vi "Set Information.vi"(8 "error in (no error)":errorcluster, 10 "Inforamtion":string="Processing......", 11 "UI_ProgressBar in":refnum<class "UI_ProgressDlg.lvclass">) -> (0 "error out":errorcluster, 3 "UI_ProgressBar out":refnum<class "UI_ProgressDlg.lvclass">)   [LabVIEW 2014, in "UI_ProgressDlg.lvlib" / "UI_ProgressDlg.lvclass"]
uses:
  UI_ProgressDlg.lvclass
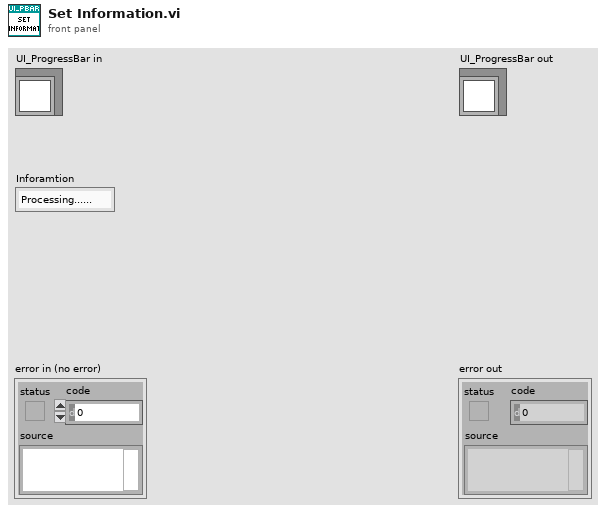
[diagram p1: front panel]
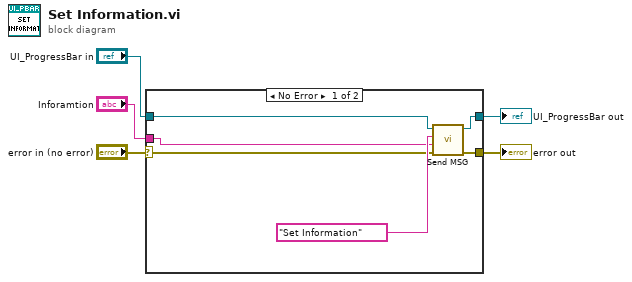
[diagram p0: block diagram]
diagram:
  n1 = case shown="No Error" "error in (no error)" {
    selector: "error in (no error)" -> [w6 w13]
    tunnel: [w10 w13] -> w4
    tunnel: [w11 w12] -> w2
    tunnel: "UI_ProgressBar in" -> [w9 w12]
    tunnel: "Inforamtion" -> [w7 _]
    frame No Error {
      n2 = call "Send MSG.vi"("error in (no error)"=w6, "msg value"=w7, "msg"="Set Information" ("Inforamtion"), "UI_ProgressBar in"=w9) -> ("error out"=w10:errorcluster, "UI_ProgressBar out"=w11:refnum<class "UI_ProgressDlg.lvclass">)  [unwired: 6 in]
    }
    frame Error {
    }
  }
  "error out" <- w4
  "UI_ProgressBar out" <- w2
